vi "get tag by name.vi"(8 "error in":errorcluster, 10 "tag":string, 11 "tag collection in":refnum<class "data bus tag collection.lvclass">) -> (0 "error out":errorcluster, 1 "located tag":refnum<class "data bus tag description.lvclass">, 3 "tag collection out":refnum<class "data bus tag collection.lvclass">)   [LabVIEW 2013, in "data bus tag collection.lvclass"]
uses:
  data bus tag collection.lvclass
  tag/data bus tag description.lvclass
  data bus tag collection.lvclass/data bus tag collection.ctl
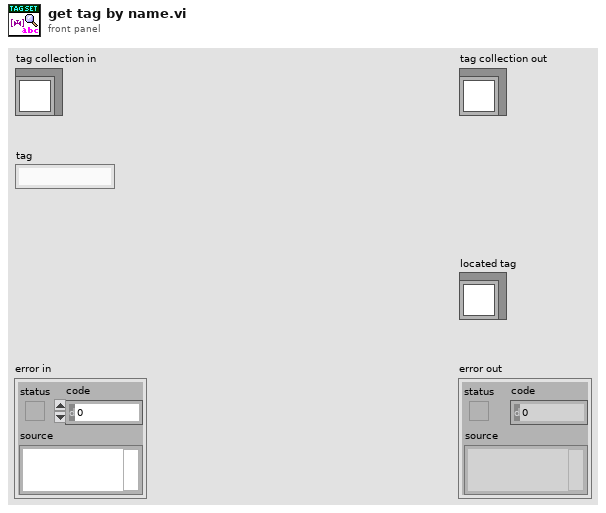
[diagram p1: front panel]
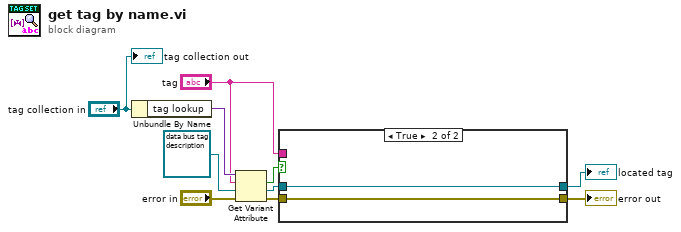
[diagram p0: block diagram]
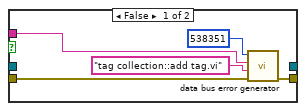
[diagram p2: hidden frame]
diagram:
  n1 = Unbundle By Name("tag collection in") -> ("tag lookup"=w5:variant)
  n2 = Get Variant Attribute(Variant=w5, name="tag", default value (empty Variant)=refnum<class "data bus tag description.lvclass"> refnum ("located tag 2"), error in="error in") -> (found=w1:bool, value=w2:refnum<class "data bus tag description.lvclass">, error out=w6:errorcluster)  [unwired: 1 out]
  n3 = case shown="True" w1 {
    tunnel: [w14 w17] -> w8
    tunnel: w6 -> [w15 w17]
    tunnel: "tag" -> [w11 _]
    tunnel: [_ w16] -> w7
    tunnel: w2 -> [_ w16]
    frame False {
      n4 = call "data bus error generator.vi"("error in"=w15, "source"="tag collection::add tag.vi", "append error message"=w11, "error code (0)"=538351) -> ("error out"=w14:errorcluster)  [unwired: 5 in]
    }
    frame True {
    }
  }
  "error out" <- w8
  "located tag" <- w7
  "tag collection out" <- "tag collection in"
